vi "PopulateEventLog.vi"(6 "max rows":i32, 7 "Listbox":refnum<vi>, 8 "error in":errorcluster, 9 "Additional Information":string, 10 "Module ID":i32, 11 "Module Name":string) -> (0 "error out":errorcluster, 1 "Additional Info OUT":string, 3 "Module Name OUT":string)   [LabVIEW 2022 SP3, in "Event Manager.lvlib"]
doc: "<b>Note:</b> This VI was modified by the <b>Validate DQMH Module</b> tool to turn off automatic error handling.\n\n____\nHAMPEL SOFTWARE ENGINEERING v2.6.0 (2023-12-19 10:54)"
uses:
  Event Manager.lvlib
  <vilib>/Utility/error.llb/Trim Whitespace One-Sided.vi
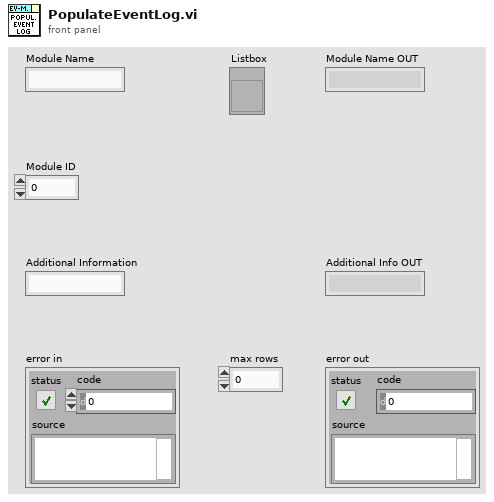
[diagram p1: front panel]
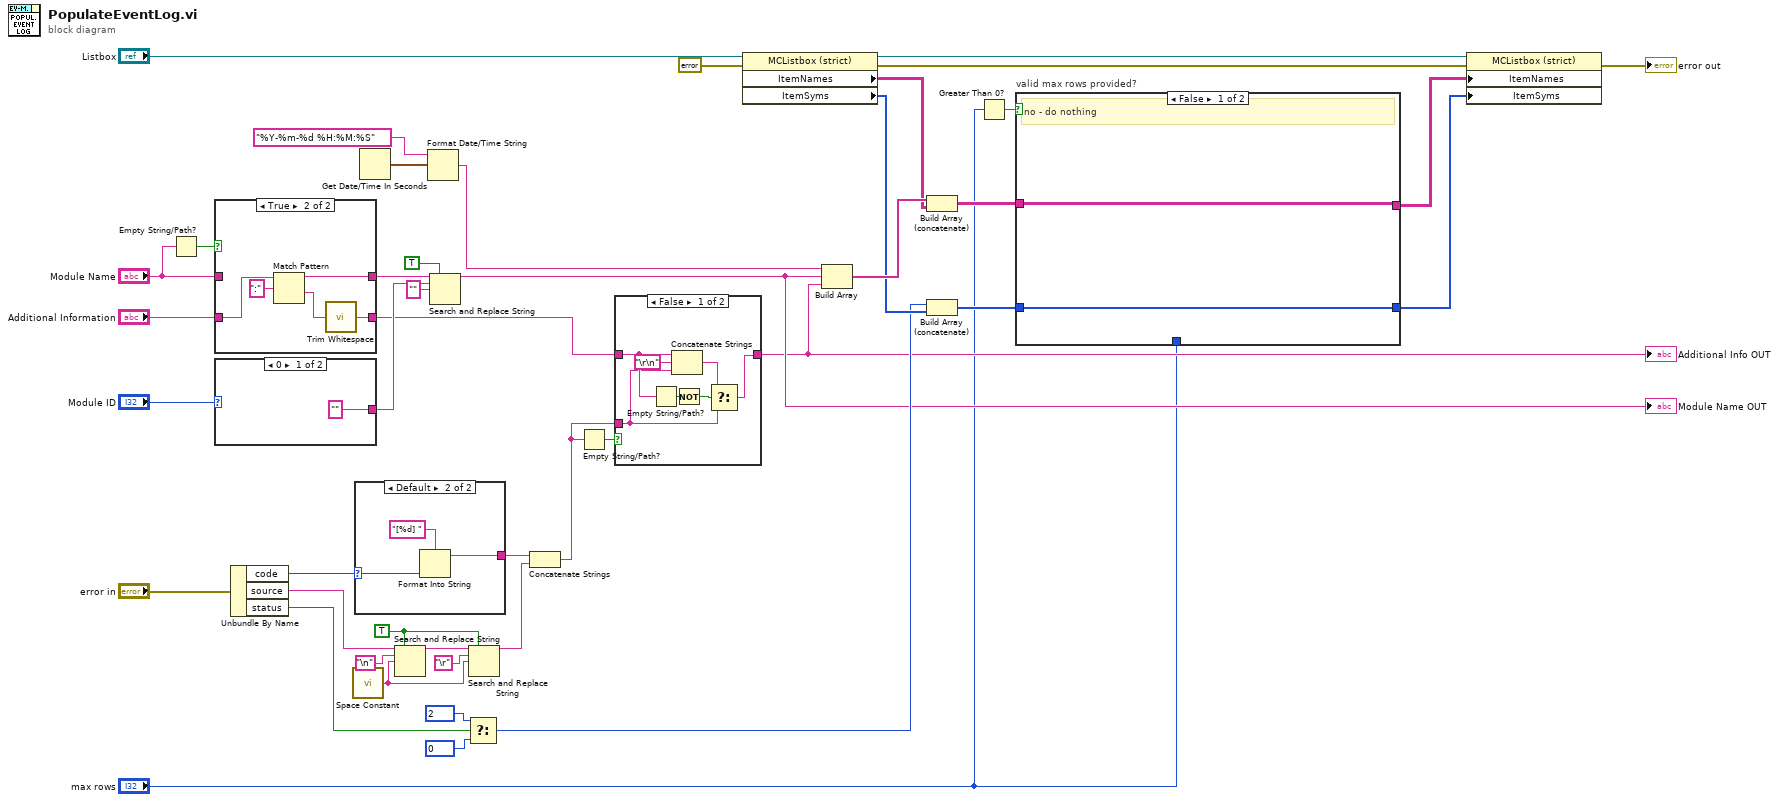
[diagram p0: block diagram]
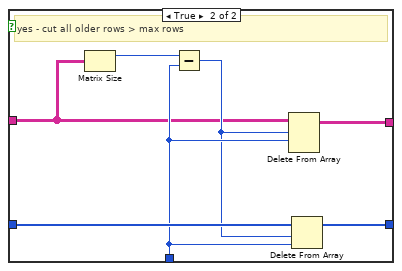
[diagram p2: hidden frame]
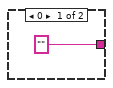
[diagram p5: hidden frame]
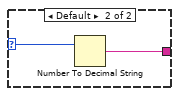
[diagram p6: hidden frame]
diagram:
  w17 = TRUE ("replace all? (F)")
  n1 = Empty String/Path?(string/path="Module Name") -> (empty?=w27:bool)
  n2 = case shown="True" w27 {
    tunnel: "Module Name" -> [w46 _]
    tunnel: "Additional Information" -> [w45 w51]
    tunnel: [w46 w49] -> w21
    tunnel: [w45 w47] -> w9
    frame False {
    }
    frame True {
      n3 = Match Pattern(string=w51, regular expression=":") -> (before substring=w49:string, after substring=w48:string)  [unwired: 1 in, 2 out]
      n4 = call <vilib>:"Trim Whitespace.vi"("string"=w48) -> ("trimmed string"=w47:string)  [unwired: 1 in]
    }
  }
  n5 = case shown="0" "Module ID" {
    selector: "Module ID" -> [_ w53]
    tunnel: ["" w54] -> w24
    frame 0 {
    }
    frame Default {
      n6 = Number To Decimal String(number=w53) -> (decimal integer string=w54:string)  [unwired: 1 in]
    }
  }
  n7 = Unbundle By Name("error in") -> ("code"=w28:i32, "source"=w19:string, "status"=w32:bool)
  n8 = call <vilib>:"Space Constant.vi"() -> ("String"=w14:string)
  n9 = case shown="Default" w28 {
    selector: w28 -> [_ w58]
    tunnel: ["" w56] -> w13
    frame 0 {
    }
    frame Default {
      n10 = Format Into String(format string="[%d] ", w58) -> (resulting string=w56:string)  [unwired: 2 in, 1 out]
    }
  }
  n11 = Get Date/Time In Seconds() -> (seconds since 1Jan1904=w40:timestamp)
  n12 = Search and Replace String(replace all?=w17, input string=w19, search string="\n", replace string=w14) -> (result string=w18:string)  [unwired: 4 in, 3 out]
  n13 = Format Date/Time String(time format string (%c)="%Y-%m-%d %H:%M:%S", seconds (now)=w40) -> (date/time string=w36:string)  [unwired: 1 in]
  n14 = Search and Replace String(replace all?=TRUE ("replace all? (F)"), input string=w21, search string=w24, replace string="" ("replace string (\"\")")) -> (result string=w20:string)  [unwired: 4 in, 3 out]
  "Module Name OUT" <- w20
  n15 = Select(t=2, s=w32, f=0) -> (s? t:f=w31:i32)
  n16 = Search and Replace String(replace all?=w17, input string=w18, search string="\r", replace string=w14) -> (result string=w12:string)  [unwired: 4 in, 3 out]
  n17 = Concatenate Strings(w13, w12) -> (w10:string)
  n18 = Empty String/Path?(string/path=w10) -> (empty?=w11:bool)
  n19 = case shown="False" w11 {
    tunnel: w10 -> [w60 _]
    tunnel: w9 -> [w62 w66]
    tunnel: [w63 w66] -> w8
    frame False {
      n20 = Empty String/Path?(string/path=w62) -> (empty?=w65:bool)
      n21 = Concatenate Strings(w62, "\r\n", w60) -> (w61:string)
      n22 = Not(x=w65) -> (.not. x?=w64:bool)
      n23 = Select(t=w61, s=w64, f=w60) -> (s? t:f=w63:string)
    }
    frame True {
    }
  }
  "Additional Info OUT" <- w8
  n24 = property on="Property Node" class="MCListbox (strict)"(reference="Listbox", error in=errorcluster {"status"=FALSE, "code"=0, "source"=""} ("error in (no error)")) -> (reference out=w38:refnum<vi>, error out=w42:errorcluster, "ItemNames"=w7:string[][], "ItemSyms"=w33:i32[])
  n25 = Build Array(w36, w20, w8) -> (w34:string[])
  n26 = Build Array (concatenate)(w34, w7) -> (w3:string[][])
  n27 = Build Array (concatenate)(w31, w33) -> (w5:i32[])
  n28 = Greater Than 0?(x="max rows") -> (x > 0?=w2:bool)
  n29 = case "valid max rows provided?" shown="False" w2 {
    tunnel: [w68 w74] -> w6
    tunnel: w5 -> [w67 w73]
    tunnel: "max rows" -> [_ w72]
    tunnel: [w67 w70] -> w4
    tunnel: w3 -> [w68 w69]
    frame False {
      # "no - do nothing"
    }
    frame True {
      # "yes - cut all older rows > max rows"
      n30 = Matrix Size(0:w69) -> (1:w75:i32)  [unwired: 1 out]
      n31 = Subtract(x=w75, y=w72) -> (x-y=w71:i32)
      n32 = Delete From Array(array=w69, length=w71, index (row)=w72) -> (array with subset deleted=w74:string[][])  [unwired: 1 in, 1 out]
      n33 = Delete From Array(array=w73, length=w71, index=w72) -> (array with subset deleted=w70:i32[])  [unwired: 1 out]
    }
  }
  n34 = property on="Property Node" class="MCListbox (strict)"(reference=w38, error in=w42, "ItemNames"=w6, "ItemSyms"=w4) -> (error out=→"error out":errorcluster)  [unwired: 1 out]
